vi "Measure Frequency.vi"() -> ()   [LabVIEW 2020]
uses:
  <vilib>/DAQmx/read.llb/DAQmx Read (Counter 1D DBL 1Chan NSamp).vi
  <vilib>/Analysis/baseanly.llb/Mean (DBL).vi
  <vilib>/DAQmx/create/channels.llb/DAQmx Create Channel (CI-Frequency).vi
  <vilib>/DAQmx/configure/timing.llb/DAQmx Timing (Implicit).vi
  <vilib>/DAQmx/miscellaneous.llb/DAQmx Fill In Error Info.vi
  <resource>/objmgr/daqmx.rc
  <vilib>/Analysis/NI_AALBase.lvlib
panel:
  in  "CI.Freq.Term":tag
  out "20 Samples Averaged":dbl
  in  "Input Wave Channel":tag
  in  "stop":bool
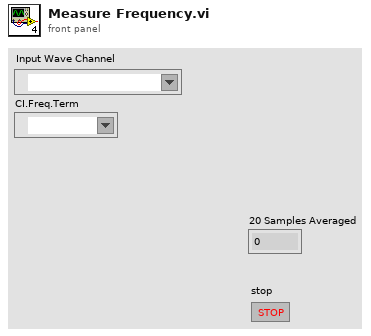
[diagram p1: front panel]
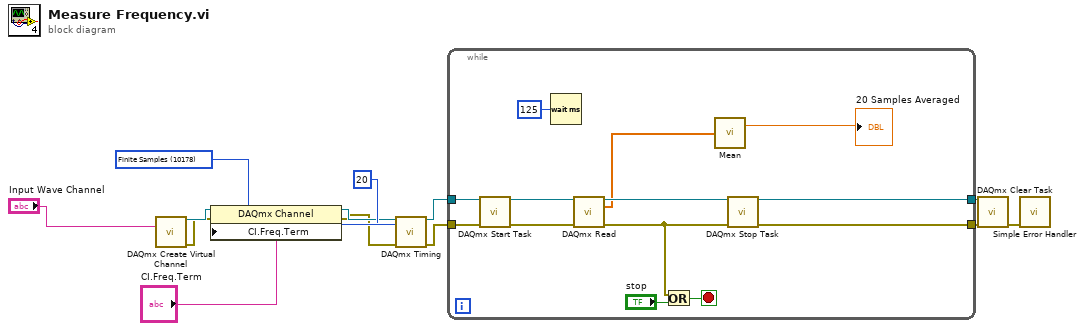
[diagram p0: block diagram]
diagram:
  w12 = 10178 items=["Finite Samples"=10178, "Continuous Samples"=10123, "Hardware Timed Single Point"=12522] ("sample mode")
  n1 = call-poly <vilib>:"DAQmx Create Virtual Channel.vi"("counter"="Input Wave Channel") -> ("task out"=w11:refnum<k21>, "error out"=w3:errorcluster)  [unwired: 13 in]
  n2 = property class="DAQmx Channel"(reference=w11, error in=w3, "CI.Freq.Term"="CI.Freq.Term") -> (reference out=w4:refnum<k21>, error out=w2:errorcluster)
  n3 = call-poly <vilib>:"DAQmx Timing.vi"("task/channels in"=w4, "sample mode"=w12, "samples per channel"=20, "error in"=w2) -> ("task out"=w7:refnum<k21>, "error out"=w6:errorcluster)  [unwired: 10 in]
  n4 = while {
    tunnel: [w23] -> w10
    tunnel: [w22] -> w9
    tunnel: w7 -> [w20]
    tunnel: w6 -> [w19]
    stop <- w25 stop-if-true
    n5 = call <vilib>:"DAQmx Start Task.vi"("task/channels in"=w20, "error in"=w19) -> ("task out"=w18:refnum<k21>, "error out"=w17:errorcluster)  [unwired: 12 in]
    n6 = Wait (ms)(milliseconds to wait=u32 125) -> ()  [unwired: 1 out]
    n7 = call-poly <vilib>:"DAQmx Read.vi"("task/channels in"=w18, "error in"=w17) -> ("task out"=w24:refnum<k21>, "data"=w15:dbl[], "error out"=w21:errorcluster)  [unwired: 11 in]
    n8 = Or(x=w21, y="stop") -> (x .or. y?=w25:bool)
    n9 = call-poly <vilib>:"Mean.vi"("X"=w15) -> ("mean"=→"20 Samples Averaged":dbl)  [unwired: 1 out]
    n10 = call <vilib>:"DAQmx Stop Task.vi"("task/channels in"=w24, "error in"=w21) -> ("task out"=w23:refnum<k21>, "error out"=w22:errorcluster)  [unwired: 12 in]
  }
  n11 = call <vilib>:"DAQmx Clear Task.vi"("task in"=w10, "error in"=w9) -> ("error out"=w8:errorcluster)  [unwired: 13 in]
  n12 = call <vilib>:"Simple Error Handler.vi"("error in (no error)"=w8) -> ()  [unwired: 4 in, 5 out]
